vi "Read.vi"(11 "Time Condition Config in":refnum<class "Time Condition Config.lvclass">) -> (2 "Elapsed":dbl, 3 "Timer":T1)   [LabVIEW 2020, in "VolatusSeqConfig.lvlib" / "Time Condition Config.lvclass"]
uses:
  Time Condition Config.lvclass
  Time Condition Config.lvclass/Time Condition Config.ctl
  Timer.ctl
  VolatusSeqConfig.lvlib
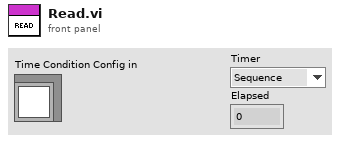
[diagram p1: front panel]
types:
  T1 = typedef "VolatusSeqConfig.lvlib/Timer.ctl" = enum16{"Sequence", "State", "Wall"}
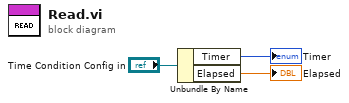
[diagram p0: block diagram]
diagram:
  n1 = Unbundle By Name("Time Condition Config in") -> ("Timer"=→"Timer":T1, "Elapsed"=→"Elapsed":dbl)
